vi "int_to_dot_separated_string.vi"(10 "integer":i32=291) -> (2 "dot fmt string":string)   [LabVIEW 2018]
doc: "Convert an integer into a dot separated string in hexadecial format e.g. convert 0x123 to 1.2.3.\n\nThe instrument returns verion numbers as hexadecimal formatted integers."
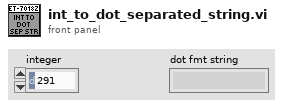
[diagram p1: front panel]
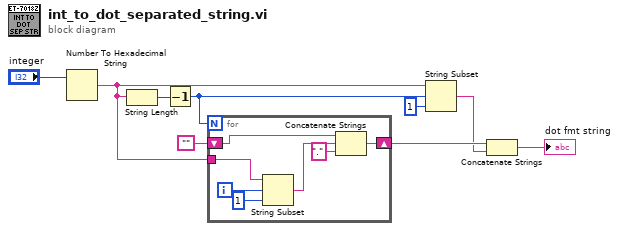
[diagram p0: block diagram]
diagram:
  n1 = Number To Hexadecimal String(2:"integer") -> (0:w7:string)  [unwired: 1 in]
  n2 = String Length(string=w7) -> (length=w6:i32)
  n3 = Decrement(x=w6) -> (x-1=w5:i32)
  n4 = for {
    N: w5 -> [_]
    tunnel: w7 -> [w10]
    shift-right: [w14] -> w3
    shift-left: "" -> [w13]
    i -> [w16]
    n5 = String Subset(string=w10, offset (0)=w16, length (rest)=1 ("length (rest)")) -> (substring=w12:string)
    n6 = Concatenate Strings(w13, w12, "." ("string")) -> (w14:string)
  }
  n7 = String Subset(string=w7, offset (0)=w5, length (rest)=1 ("length (rest)")) -> (substring=w2:string)
  n8 = Concatenate Strings(w3, w2) -> (→"dot fmt string":string)
